vi "Gamma_range.vi"(2 "Illuminant Table":string[][](array[string]), 3 "NumberOfRows":i32) -> (0 "GammaInterval":dbl[](array[numeric]), 1 "In range?":bool)   [LabVIEW 2014]
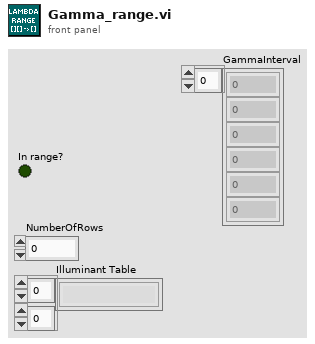
[diagram p1: front panel]
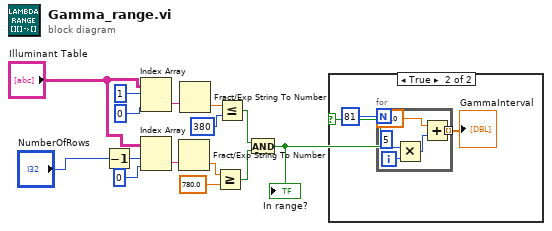
[diagram p0: block diagram]
diagram:
  n1 = Decrement(x="NumberOfRows") -> (x-1=w14:i32)
  n2 = Index Array(array="Illuminant Table", index (row)=1, index (col)=0) -> (element=w11:string)
  n3 = Index Array(array="Illuminant Table", index (row)=w14, index (col)=0 ("disabled index (col)")) -> (element=w10:string)
  n4 = Fract/Exp String To Number(string=w10) -> (number=w8:dbl)  [unwired: 3 in, 1 out]
  n5 = Fract/Exp String To Number(string=w11) -> (number=w5:dbl)  [unwired: 3 in, 1 out]
  n6 = Greater Or Equal?(x=w8, y=780.0) -> (x >= y?=w2:bool)
  n7 = Less Or Equal?(x=w5, y=380 ("x")) -> (x <= y?=w3:bool)
  n8 = And(x=w3, y=w2) -> (x .and. y?=w6:bool)
  "In range?" <- w6
  n9 = case shown="True" w6 {
    frame False {
    }
    frame True {
      n10 = for {
        N: 81 -> [_]
        tunnel: [w19] -> w17 mode=indexing
        i -> [w21]
        n11 = Multiply(x=5, y=w21) -> (x*y=w22:i32)
        n12 = Add(x=380.0, y=w22) -> (x+y=w19:dbl)
      }
      "GammaInterval" <- w17
    }
  }
